vi "sub_NMEA-LatLon.vi"(10 "nmea sel":string="$GNGGA", 11 "gnss str":string) -> (2 "latlong":cluster{"Lat":dbl, "Long":dbl} {"Lat" format="%.7f"; "Long" format="%.7f"}, 3 "val":bool)   [LabVIEW 2019]
uses:
  NMEA_v1.1/NMEA_GPGGA-data.ctl
  NMEA_v1.1/NMEA_LatitudeDirection.ctl
  NMEA_v1.1/NMEA_LongitudeDirection.ctl
  NMEA_v1.1/NMEA_GPS-Quality.ctl
  Ctrl/cmd_common.ctl
  NMEA_v1.1/NMEA.lvlib
panel:
  out "$GPGGA-message_OUT":T1={"TimeStamp"=timestamp(0 s since 1904-01-01), "Latitude"=0.0, "Latitude-Direction"=enum."", "Longitude"=1.0, "Longitude-Direction"=enum."", "GPS-Quality"=enum."GPS fix (SPS)", "Number of Satellites"=0, "Horizontal Dilution of Precision"=0.0, "Altitude above Mean-Sea-Level"=0.0, "Geoidal separation"=0.0, "Time since last DGPS update"=0.0, "DGPS reference station ID"=0} {"Time since last DGPS update" format="%.02f [s]"; "Geoidal separation" format="%.02f [m]"; "Altitude above Mean-Sea-Level" format="%.02f [m]"; "Horizontal Dilution of Precision" format="%.02f [HDOP]"; "Longitude" format="%0.4f [long]"; "Latitude" format="%.04f [lat]"; "TimeStamp" format="%<%.2X>T"}
  out "nmea protocol":string[](array[string])
  out "gnss str 2":string
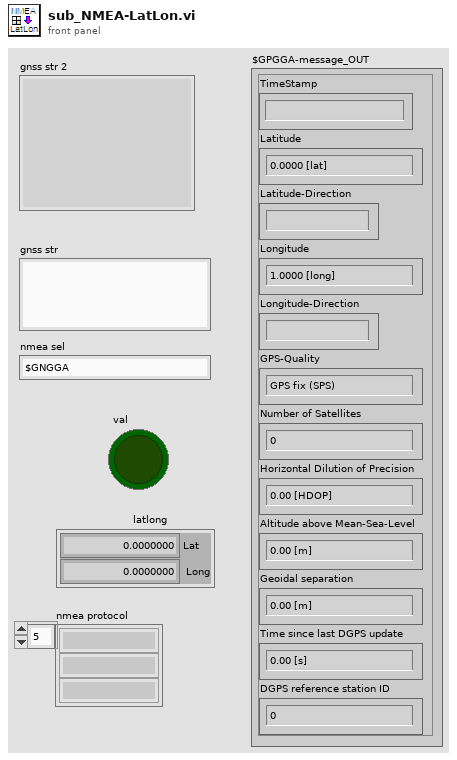
[diagram p1: front panel]
types:
  T1 = typedef "NMEA.lvlib/NMEA_GPGGA-data.ctl" = cluster{"TimeStamp":timestamp, "Latitude":dbl, "Latitude-Direction":T2, "Longitude":dbl, "Longitude-Direction":T3, "GPS-Quality":T4, "Number of Satellites":i32, "Horizontal Dilution of Precision":dbl, "Altitude above Mean-Sea-Level":dbl, "Geoidal separation":dbl, "Time since last DGPS update":dbl, "DGPS reference station ID":i32}
  T2 = typedef "NMEA.lvlib/NMEA_LatitudeDirection.ctl" = enum16{"", "North", "South"}
  T3 = typedef "NMEA.lvlib/NMEA_LongitudeDirection.ctl" = enum16{"", "East", "West"}
  T4 = typedef "NMEA.lvlib/NMEA_GPS-Quality.ctl" = enum16{"Invalid", "GPS fix (SPS)", "DGPS fix", "PPS fix", "Real Time Kinematic", "Float RTK", "estimated", "Manual input mode", "Simulation mode"}
  T5 = typedef "cmd_common.ctl" = enum16{"read", "write"}
  T6 = cluster{"lat_index":i32, "lon_index":i32, "heading index":i32}
  T7 = cluster{"$GPGGA-message_OUT":cluster{"TimeStamp":timestamp, "Latitude":dbl, "Latitude-Direction":T2, "Longitude":dbl, "Longitude-Direction":T3, "GPS-Quality":T4, "N of Satellites":i32, "HDOP":dbl, "Altitude above Mean-Sea-Level":dbl, "Geoidal separation":dbl, "Time since last DGPS update":dbl, "DGPS reference station ID":i32}}
  T8 = typedef "ublox-ui_main.ctl" = cluster{"Latitude":dbl, "Longitude":dbl, "Fix Mode":string, "3D Acc.m":dbl, "2D Acc.m":dbl, "PDOP":dbl, "HDOP":dbl}
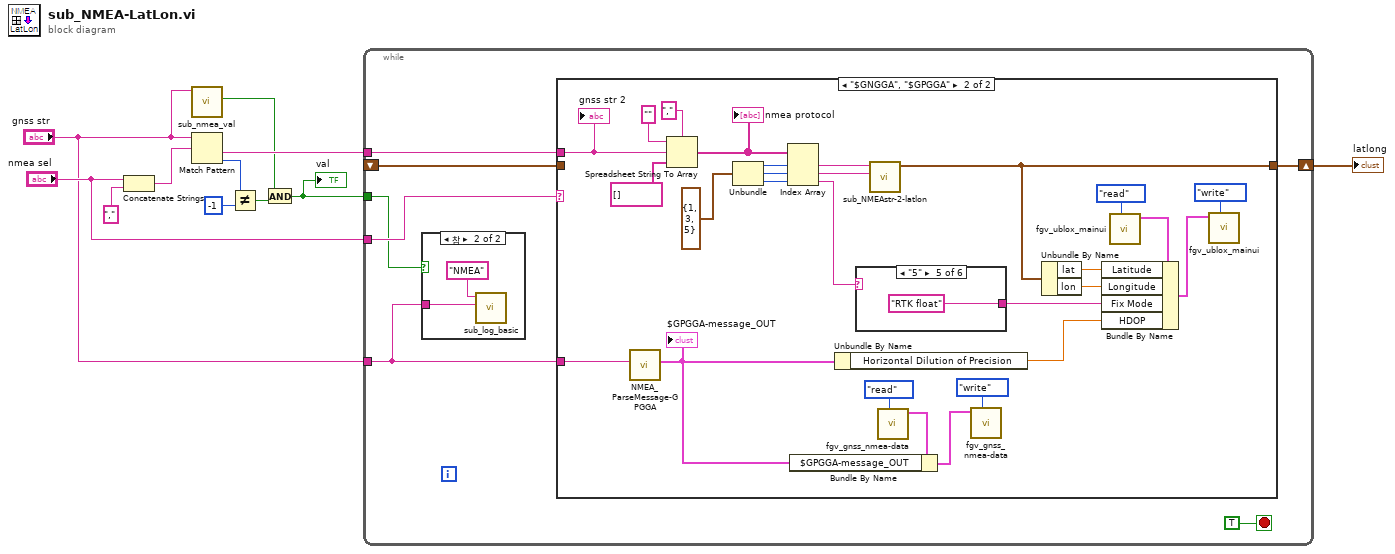
[diagram p0: block diagram]
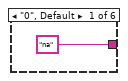
[diagram p4: hidden frame]
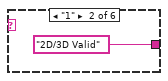
[diagram p5: hidden frame]
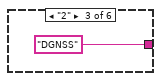
[diagram p6: hidden frame]
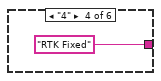
[diagram p7: hidden frame]
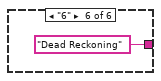
[diagram p8: hidden frame]
diagram:
  n1 = Concatenate Strings("nmea sel", "," ("문자열")) -> (w6:string)
  n2 = call "sub_nmea_val.vi"("nmea str"="gnss str") -> ("checksum"=w4:bool)  [unwired: 9 in, 1 out]
  n3 = Match Pattern(string="gnss str", regular expression=w6) -> (after substring=w9:string, offset past match=w11:i32)  [unwired: 1 in, 2 out]
  n4 = Not Equal?(x=w11, y=-1) -> (x != y?=w5:bool)
  n5 = And(x=w4, y=w5) -> (x .and. y?=w3:bool)
  "val" <- w3
  n6 = while {
    tunnel: w3 -> [w12]
    shift-right: [w17] -> w8
    shift-left: _ -> [w16]
    tunnel: w9 -> [w15]
    tunnel: "nmea sel" -> [w14]
    tunnel: "gnss str" -> [w13]
    stop <- TRUE stop-if-true
    n7 = case shown="참" w12 {
      tunnel: w13 -> [_ w19]
      frame False {
      }
      frame True {
        n8 = call "sub_log_basic.vi"("desc"=w19, "Title"="NMEA") -> ()  [unwired: 9 in, 1 out]
      }
    }
    n9 = case shown="\"$GNGGA\", \"$GPGGA\"" w14 {
      tunnel: [w21 w30] -> w17
      tunnel: w16 -> [w21 _]
      tunnel: w15 -> [_ w31]
      tunnel: w13 -> [_ w32]
      frame "거짓", Default {
      }
      frame "$GNGGA", "$GPGGA" {
        n10 = call "NMEA_ParseMessage-GPGGA.vi"("$GPGGA-message_IN"=w32) -> ("$GPGGA-message_OUT"=w23:T1)  [unwired: 9 in, 1 out]
        "$GPGGA-message_OUT" <- w23
        n11 = Spreadsheet String To Array(delimiter (Tab)="," ("구분 문자 (탭)"), format string="" ("포맷 문자열"), spreadsheet string=w31, array type (2D Dbl)=string[] []) -> (array=w44:string[])
        "nmea protocol" <- w44
        n12 = Unbundle(T6 {"lat_index"=1, "lon_index"=3, "heading index"=5} ("index cluster")) -> ("lat_index"=w42:i32, "lon_index"=w43:i32, "heading index"=w41:i32)
        n13 = Index Array(array=w44, index #1=w42, index #2=w43, index #3=w41) -> (element #1=w48:string, element #2=w35:string, element #3=w33:string)
        n14 = Unbundle By Name(w23) -> ("Horizontal Dilution of Precision"=w27:dbl)
        n15 = case shown="\"5\"" w33 {
          tunnel: ["na" "2D/3D Valid" "DGNSS" "RTK Fixed" "RTK float" "Dead Reckoning"] -> w34
          frame "0", Default {
          }
          frame "1" {
          }
          frame "2" {
          }
          frame "4" {
          }
          frame "5" {
          }
          frame "6" {
          }
        }
        n16 = call "sub_NMEAstr-2-latlon.vi"("문자열"=w35, "문자열 2"=w48) -> ("LatLon"=w30:cluster{"lat":dbl, "lon":dbl})  [unwired: 9 in]
        n17 = call "fgv_gnss_nmea-data.vi"("cmd"=cmd_common."read") -> ("nmea-data out"=w24:T7)  [unwired: 10 in]
        n18 = Bundle By Name(cluster=w24, "$GPGGA-message_OUT"=w23) -> (w22:T7)
        n19 = call "fgv_gnss_nmea-data.vi"("cmd"=cmd_common."write", "nmea-data"=w22) -> ()  [unwired: 9 in, 1 out]
        n20 = Unbundle By Name(w30) -> ("lat"=w28:dbl, "lon"=w29:dbl)
        n21 = call "fgv_ublox_mainui.vi"("cmd"=cmd_common."read") -> ("MainUI gnss out"=w37:T8)  [unwired: 10 in]
        n22 = Bundle By Name(cluster=w37, "Latitude"=w28, "Longitude"=w29, "Fix Mode"=w34, "HDOP"=w27) -> (w36:T8)
        n23 = call "fgv_ublox_mainui.vi"("cmd"=cmd_common."write", "MainUI gnss"=w36) -> ()  [unwired: 9 in, 1 out]
        "gnss str 2" <- w31
      }
    }
  }
  "latlong" <- w8
